vi "Revert & Restat _VM.vi"(0 "VM Name":string, 1 "Basic input cammand":string="perl vmware-cmd.pl -H 10.164.43.31 -U root -P INpwdAdm!n \"", 2 "Sefix Like Softe rest/\" revertsnapshot":string="\" revertsnapshot", 3 "error in (no error)":errorcluster, 4 "Basic  vSphere Path":path=path "C:/Program Files (x86)/VMware/VMware vSphere CLI/bin", 8 "VM's path":path) -> (5 "standard output":string, 6 "standard error":string, 7 "concatenated Cammand":string, 10 "error out":errorcluster)   [LabVIEW 2015]
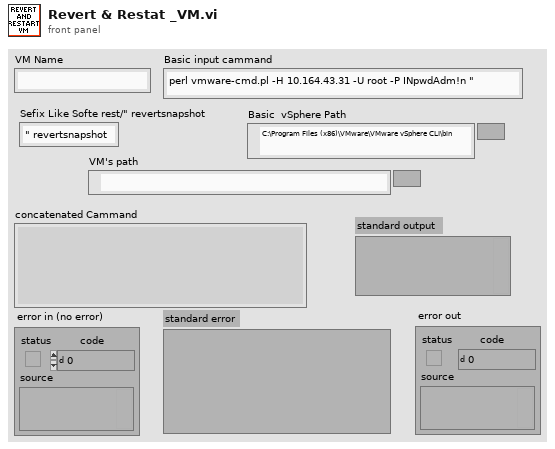
[diagram p1: front panel]
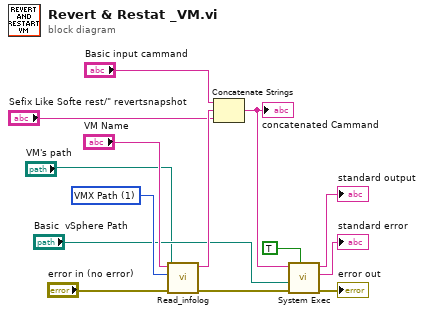
[diagram p0: block diagram]
diagram:
  w9 = u16 1 items=["VM Name", "VMX Path", "OS Detail", "OS Bitness"] ("Ring")
  n1 = call "Read_infolog.vi"("vm name"="VM Name", "Details of vm"=w9, "VM's path"="VM's path", "error in"="error in (no error)") -> ("VMX Path details"=w8:string, "error out"=w3:errorcluster)  [unwired: 5 in]
  n2 = Concatenate Strings("Basic input cammand", w8, "Sefix Like Softe rest/\" revertsnapshot") -> (w12:string)
  "concatenated Cammand" <- w12
  n3 = call <vilib>:"System Exec.vi"("wait until completion? (T)"=TRUE, "error in (no error)"=w3, "working directory"="Basic  vSphere Path", "command line"=w12) -> ("error out"=→"error out":errorcluster, "standard error"=→"standard error":string, "standard output"=→"standard output":string)  [unwired: 4 in, 1 out]
